vi "Clear Hardware.vi"(2 "error in (no error)":errorcluster, 3 "LTA-HS in":refnum<class "LTA-HS.lvclass">) -> (0 "error out":errorcluster, 1 "LTA-HS out":refnum<class "LTA-HS.lvclass">)   [LabVIEW 2013, in "LTA-HS.lvclass"]
doc: "This VI resets any necessary hardware so that the device will be ready for the next run."
uses:
  LTA-HS.lvclass
  Device/Device.lvclass
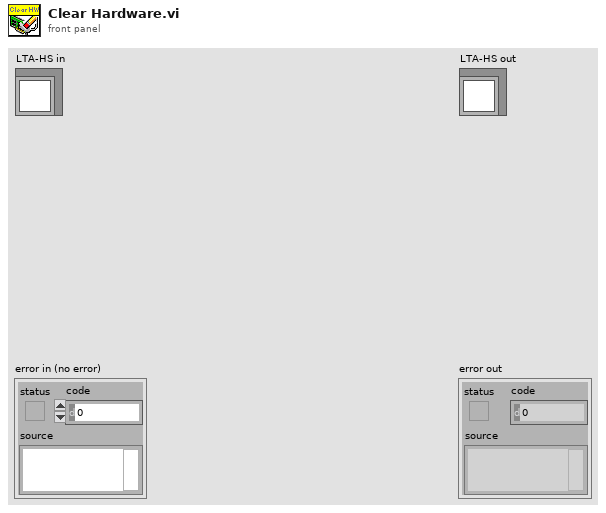
[diagram p1: front panel]
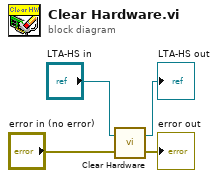
[diagram p0: block diagram]
diagram:
  n1 = call-parent "Clear Hardware.vi"("error in (no error)"="error in (no error)", "Device in"="LTA-HS in") -> ("error out"=→"error out":errorcluster, "Device out"=→"LTA-HS out":refnum<class "LTA-HS.lvclass">)
